vi "GTH.Comm.vi"(8 "Error In":errorcluster caption="错误输入", 10 "SCPI CMD":string, 11 "USB Port In":refnum<visa-resource-name>) -> (0 "Error Out":errorcluster caption="错误输出", 1 "OK?":bool, 2 "Return":string, 3 "USB Port Out":refnum<visa-resource-name>, 4 "Recv Length":u32, 5 "Send Length":u32)   [LabVIEW 2012, in "Lib_UEL.ATE.lvlib" / "STM32-CoreBD.lvlib"]
uses:
  STM32-CoreBD.lvlib
panel:
  out "Query":bool
  # "/* IEEE Mandated Commands (SCPI std V1999.0 4.1.1) */\n    {\"*CLS\", SCPI_CoreCls,},\n    {\"*ESE\", SCPI_CoreEse,},    {\"*ESE?\", SCPI_CoreEseQ,},\n    {\"*ESR?\", SCPI_CoreEsrQ,},\n    {\"*IDN?\", SCPI_CoreIdnQ,},\n    {\"*OPC\", SCPI_CoreOpc,},    {\"*OPC?\", SCPI_CoreOpcQ,},\n    {\"*RST\", SCPI_CoreRst,},\n    {\"*SRE\", SCPI_CoreSre,},    {\"*SRE?\", SCPI_CoreSreQ,},\n    {\"*STB?\", SCPI_CoreStbQ,},\n    {\"*TST?\", SCPI_CoreTstQ,},\n    {\"*WAI\", SCPI_CoreWai,},\n\n    /* Required SCPI commands (SCPI std V1999.0 4.2.1) */\n    {\"SYSTem:ERRor[:NEXT]?\", SCPI_SystemErrorNextQ,},\n    {\"SYSTem:ERRor:COUNt?\", SCPI_SystemErrorCountQ,},\n    {\"SYSTem:VERSion?\", SCPI_SystemVersionQ,},\n\n    {\"STATus:QUEStionable[:EVENt]?\", SCPI_StatusQuestionableEventQ,},\n    {\"STATus:QUEStionable:ENABle\", SCPI_StatusQuestionableEnable,},\n    {\"STATus:QUEStionable:ENABle?\", SCPI_StatusQuestionableEnableQ,},\n\n    {\"STATus:PRESet\", SCPI_StatusPreset,},,\n\t\n\t/*CUSTOM*/\n\t\n\t{\"MEASure:VMAX?\", GTH_MeasureVMAXQ,},\n\t{\"MEASure:VMIN?\", GTH_MeasureVMINQ,},\n\t{\"MEASure:VPP?\", GTH_MeasureVPPQ,},\n\t{\"MEASure:VRMS?\", GTH_MeasureVRMSQ,},\n\t{\"MEASure:VAVerage?\", GTH_MeasureVaverageQ,},\n\t{\"MEASure:FREQuency?\", GTH_MeasureFrequencyQ,},\t\n\t{\"MEASure:SET:AMPlification\", GTH_MeasureSetAmp,},\n\t\n\t{\"TIMebase:SAMPlerate\", GTH_TimebaseSamplerate,},\n\t\n\t{\"WAVeform:DATA?\", GTH_WaveformDataQ,},\n\t\n\t{\"DISPlay:TEXT\", GTH_DisplayText,},\n\t{\"DISPlay:TEXT:CLEar\", GTH_DisplayTextClear,},\n\t\n\t{\"CONFigure:RELay\", GTH_ConfigureRelay,},\n\t{\"CONFigure:USB:RET\", GTH_ConfigureUSBRST,},\n\t\n\t{\"APPLy:SINusoid\", GTH_ApplySinusoid,},\n\t{\"APPLy:WAV\", GTH_ApplyWAV,},\n\t{\"APPLy:ONCHip\", GTH_ApplyOnchip,},\n\t\n\t{\"OUTPut\", GTH_Output,},\n\t\n    {\"TEST:BOOL\", TEST_Bool,},\n    {\"TEST:CHOice?\", TEST_ChoiceQ,},\n    {\"TEST#:NUMbers#\", TEST_Numbers,},"
  # "SYST:ERR:COUNT?\n*CLS\nCONF:EEP:WRITE 1,\"2015-08-12,B2,4.0,4.0\"\nAPPL:ONCH"
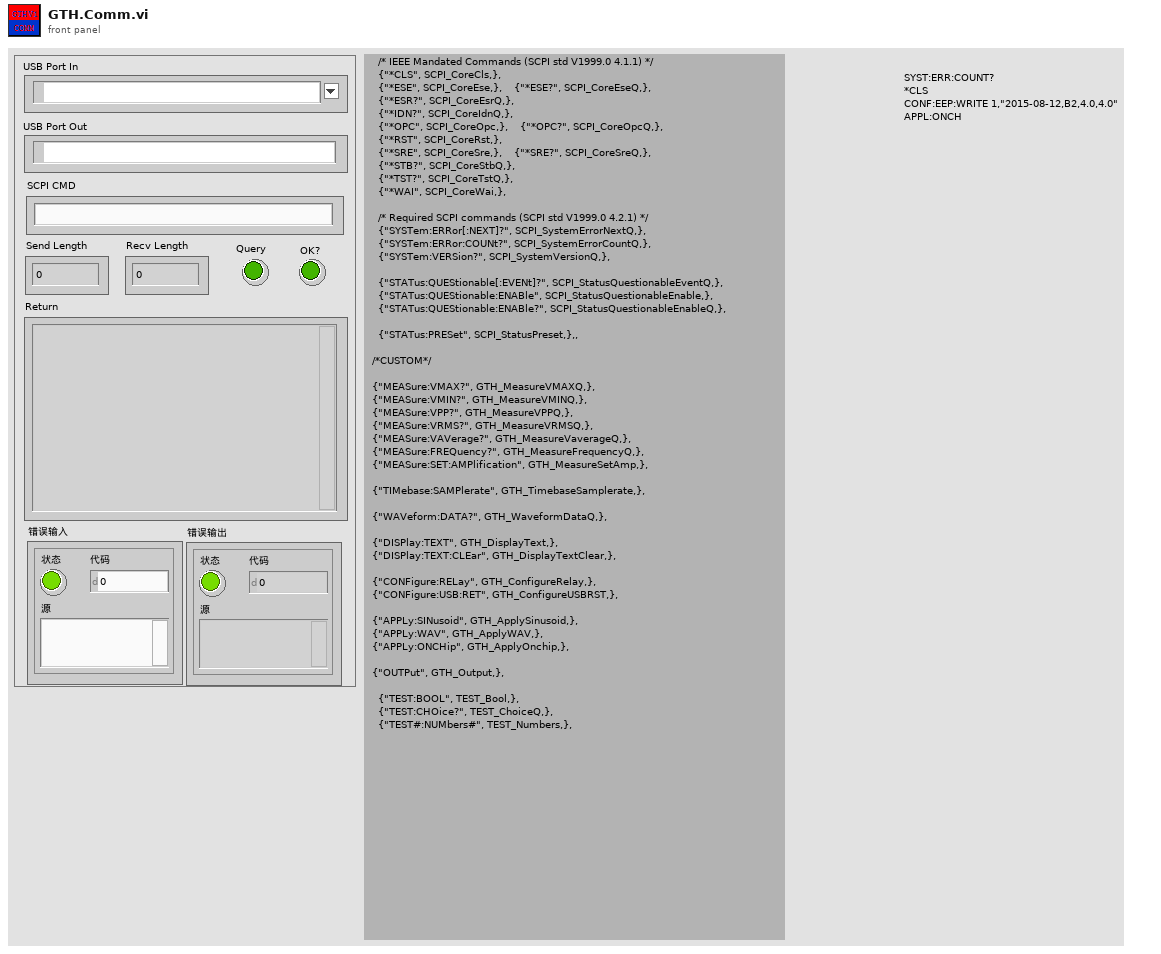
[diagram p1: front panel]
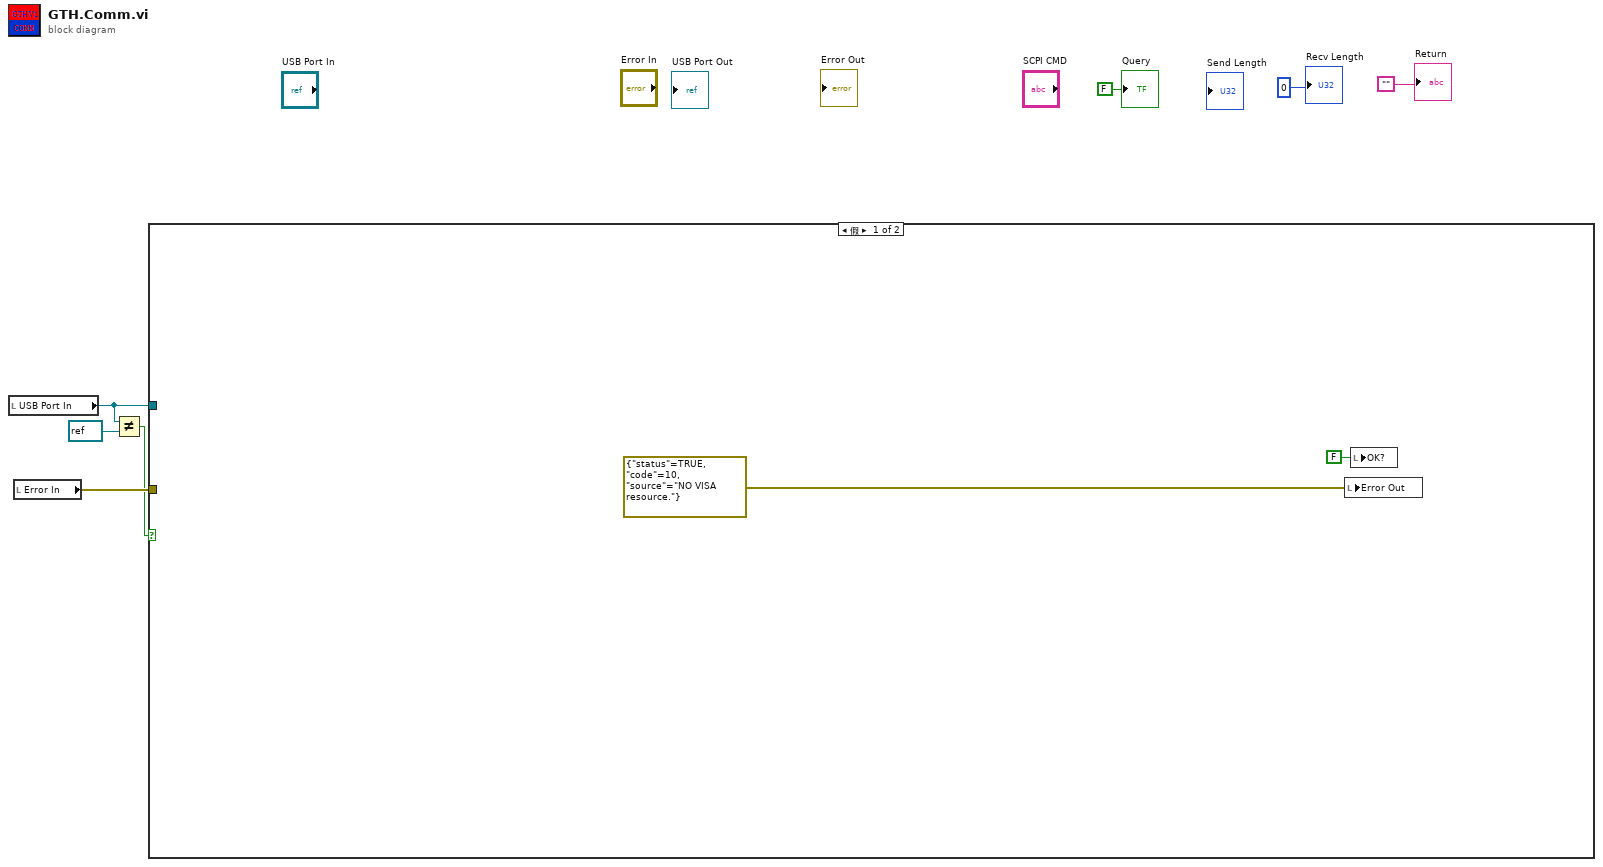
[diagram p0: block diagram]
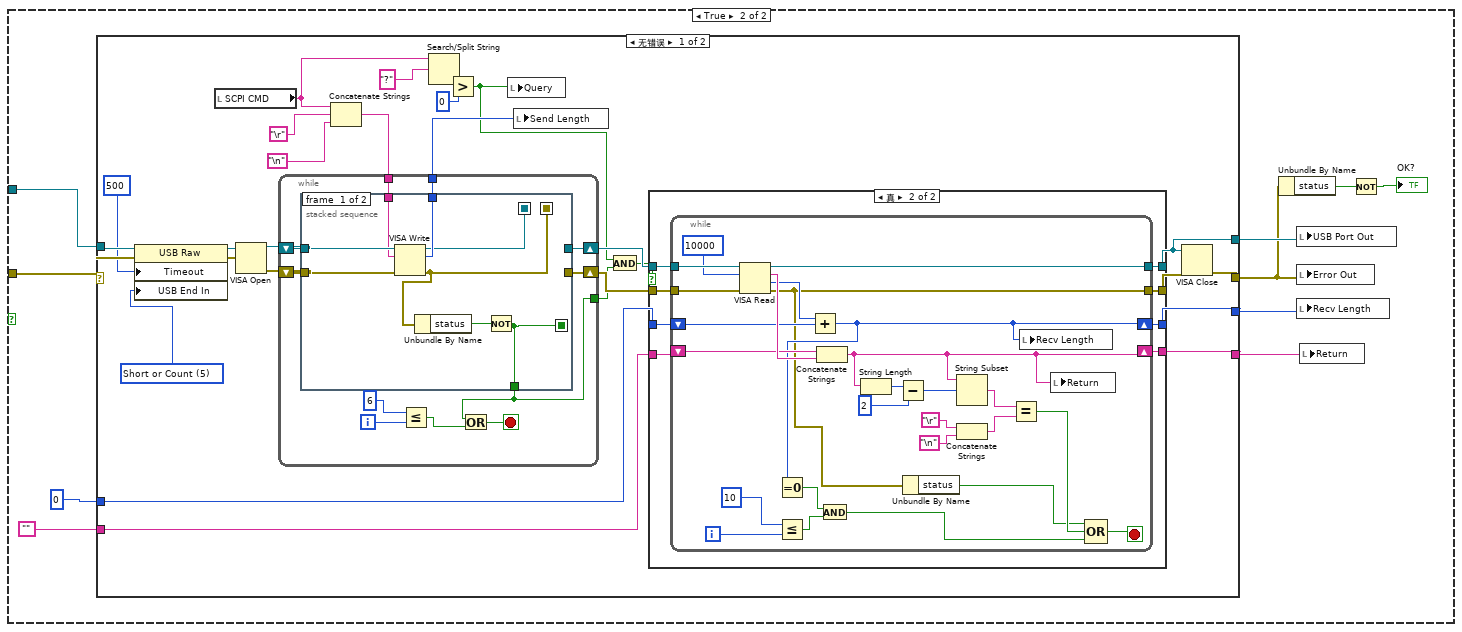
[diagram p2: hidden frame]
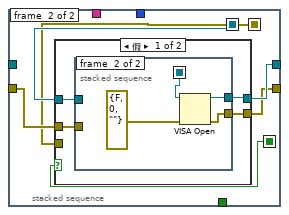
[diagram p3: hidden frame]
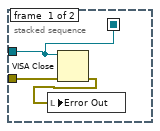
[diagram p4: hidden frame]
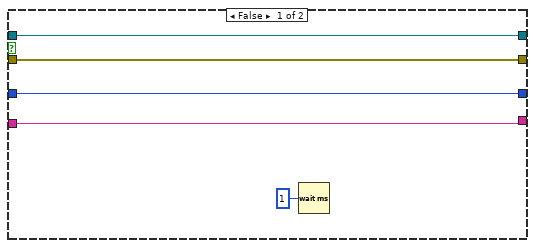
[diagram p6: hidden frame]
diagram:
  n1 = local read "USB Port In"() -> (w3:refnum<visa-resource-name>)
  n2 = local read "Error In"() -> (w7:errorcluster)
  n3 = Not Equal?(x=w3, y=refnum<visa-resource-name> refnum) -> (x != y?=w1:bool)
  n4 = case shown="假" w1 {
    tunnel: w7 -> [_ w19]
    tunnel: w3 -> [_ w10]
    frame False {
      n5 = local write "Error Out"(errorcluster {"status"=TRUE, "code"=10, "source"="NO VISA resource."} ("Error Out")) -> ()
      n6 = local write "OK?"(FALSE ("OK?")) -> ()
    }
    frame True {
      n7 = case shown="无错误" w19 {
        selector: w19 -> [w28 w128]
        tunnel: [w37 w128] -> w13
        tunnel: w10 -> [w29 w126]
        tunnel: "" -> [w39 w127]
        tunnel: [w23 w127] -> w14
        tunnel: [w36 w126] -> w17
        tunnel: 0 -> [w35 w125]
        tunnel: [w34 w125] -> w15
        frame No Error {
          w26 = u16 5 items=["None"=0, "Short"=4, "Short or Count"=5] ("USB Settings:End Mode for Reads")
          n8 = property class="USB Raw"(reference=w29, error in=w28, "Timeout"=u32 500 ("General Settings:Timeout Value"), "USB End In"=w26) -> (reference out=w25:refnum<visa-resource-name>, error out=w24:errorcluster)
          n9 = local read "SCPI CMD"() -> (w33:string)
          n10 = VISA Open(error in (no error)=w24, VISA resource name=w25) -> (VISA resource name=w44:refnum<visa-resource-name>, error out=w43:errorcluster)  [unwired: 3 in]
          n11 = Concatenate Strings(w33, "\r", "\n") -> (w30:string)
          n12 = while {
            tunnel: [w56] -> w42
            tunnel: w30 -> [w54]
            tunnel: [w49] -> w21
            shift-right: [w55] -> w41
            shift-left: w44 -> [w58]
            shift-right: [w53] -> w40
            shift-left: w43 -> [w57]
            i -> [w48]
            stop <- w51 stop-if-true
            n13 = stacked-sequence {
              seq-local: [w61 _] -> [_ w72]
              seq-local: [w60 _] -> [_ w69]
              seq-local: [w59 _] -> [_ w67]
              tunnel: w58 -> [w66 _]
              tunnel: w57 -> [w65 w71]
              tunnel: [w64 _] -> w56
              tunnel: [_ w70] -> w55
              tunnel: w54 -> [w63 _]
              tunnel: [_ w68] -> w53
              tunnel: [w61 _] -> w49
              frame #0 {
                n14 = VISA Write(VISA resource name=w66, write buffer=w63, error in (no error)=w65) -> (VISA resource name out=w60:refnum<visa-resource-name>, return count=w64:u32, error out=w59:errorcluster)
                n15 = Unbundle By Name(w59) -> ("status"=w62:bool)
                n16 = Not(x=w62) -> (.not. x?=w61:bool)
              }
              frame #1 {
                n17 = case shown="假" w72 {
                  tunnel: w69 -> [w75 w85]
                  tunnel: w71 -> [w76 _]
                  tunnel: [w74 w85] -> w70
                  tunnel: [w73 w84] -> w68
                  tunnel: w67 -> [_ w84]
                  frame False {
                    n18 = stacked-sequence {
                      seq-local: [w77 _] -> [_ w83]
                      tunnel: w76 -> [w79 _]
                      tunnel: w75 -> [w77 _]
                      tunnel: [_ w81] -> w74
                      tunnel: [_ w80] -> w73
                      frame #0 {
                        n19 = VISA Close(VISA resource name=w77, error in (no error)=w79) -> (error out=w78:errorcluster)
                        n20 = local write "Error Out"(w78) -> ()
                      }
                      frame #1 {
                        n21 = VISA Open(error in (no error)=errorcluster {"status"=FALSE, "code"=0, "source"=""} ("错误输入（无错误）"), VISA resource name=w83) -> (VISA resource name=w81:refnum<visa-resource-name>, error out=w80:errorcluster)  [unwired: 3 in]
                      }
                    }
                  }
                  frame True {
                  }
                }
              }
            }
            n22 = Less Or Equal?(x=6, y=w48) -> (x <= y?=w50:bool)
            n23 = Or(x=w49, y=w50) -> (x .or. y?=w51:bool)
          }
          n24 = Search/Split String(string=w33, search string/char (-)="?" ("搜索字符串/字符(-)")) -> (offset of match=w46:i32)  [unwired: 1 in, 2 out]
          n25 = Greater?(x=w46, y=0) -> (0:w22:bool)
          n26 = local write "Query"(w22) -> ()
          n27 = local write "Send Length"(w42) -> ()
          n28 = And(x=w22, y=w21) -> (x .and. y?=w20:bool)
          n29 = case shown="真" w20 {
            tunnel: w41 -> [w88 w98]
            tunnel: w40 -> [w89 w97]
            tunnel: w39 -> [w90 w96]
            tunnel: [w90 w91] -> w23
            tunnel: [w88 w95] -> w36
            tunnel: [w89 w94] -> w38
            tunnel: w35 -> [w87 w93]
            tunnel: [w87 w92] -> w34
            frame False {
              n30 = Wait (ms)(milliseconds to wait=u32 1 ("等待时间（毫秒）")) -> ()  [unwired: 1 out]
            }
            frame True {
              n31 = while {
                tunnel: w98 -> [w123]
                tunnel: w97 -> [w124]
                shift-right: [w102] -> w91
                shift-left: w96 -> [w120]
                tunnel: [w112] -> w95
                tunnel: [w100] -> w94
                shift-right: [w101] -> w92
                shift-left: w93 -> [w110]
                i -> [w109]
                stop <- w106 stop-if-true
                n32 = VISA Read(VISA resource name=w123, byte count=u32 10000 ("字节总数"), error in (no error)=w124) -> (VISA resource name out=w112:refnum<visa-resource-name>, read buffer=w121:string, return count=w111:u32, error out=w100:errorcluster)
                n33 = Less Or Equal?(x=10, y=w109) -> (x <= y?=w105:bool)
                n34 = Add(x=w111, y=w110) -> (x+y=w101:u32)
                n35 = Equal To 0?(x=w101) -> (x = 0?=w104:bool)
                n36 = Concatenate Strings(w120, w121) -> (w102:string)
                n37 = And(x=w104, y=w105) -> (x .and. y?=w103:bool)
                n38 = String Length(string=w102) -> (length=w119:i32)
                n39 = Subtract(x=w119, y=2) -> (x-y=w117:i32)
                n40 = Unbundle By Name(w100) -> ("status"=w99:bool)
                n41 = String Subset(string=w102, offset (0)=w117) -> (substring=w114:string)  [unwired: 1 in]
                n42 = Concatenate Strings("\r", "\n") -> (w113:string)
                n43 = Equal?(x=w114, y=w113) -> (x = y?=w107:bool)
                n44 = local write "Recv Length"(w101) -> ()
                n45 = local write "Return"(w102) -> ()
                n46 = Compound Arithmetic op=OR(w99, w107, w103) -> (w106:bool)
              }
            }
          }
          n47 = VISA Close(VISA resource name=w36, error in (no error)=w38) -> (error out=w37:errorcluster)
        }
        frame Error {
        }
      }
      n48 = Unbundle By Name(w13) -> ("status"=w11:bool)
      n49 = local write "USB Port Out"(w17) -> ()
      n50 = local write "Error Out"(w13) -> ()
      n51 = local write "Recv Length"(w15) -> ()
      n52 = local write "Return"(w14) -> ()
      n53 = Not(x=w11) -> (.not. x?=→"OK?":bool)
    }
  }
  "Query" <- FALSE ("Return")
  "Recv Length" <- 0
  "Return" <- ""
